vi "Get Monitor Configuration.vi"(8 "error in (no error)":errorcluster) -> (0 "error out":errorcluster, 1 "Primary Display Index":i32, 2 "Display Preview":picture, 3 "Display Areas":T1(array[cluster]))   [LabVIEW 2023]
doc: "This will return an array of clusters with the Horizontal and verticle dimensions in pixels for each display."
uses:
  <vilib>/Analysis/baseanly.llb/Mean (DBL).vi
  System.Windows.Forms
  System.Drawing
  <vilib>/Analysis/NI_AALBase.lvlib
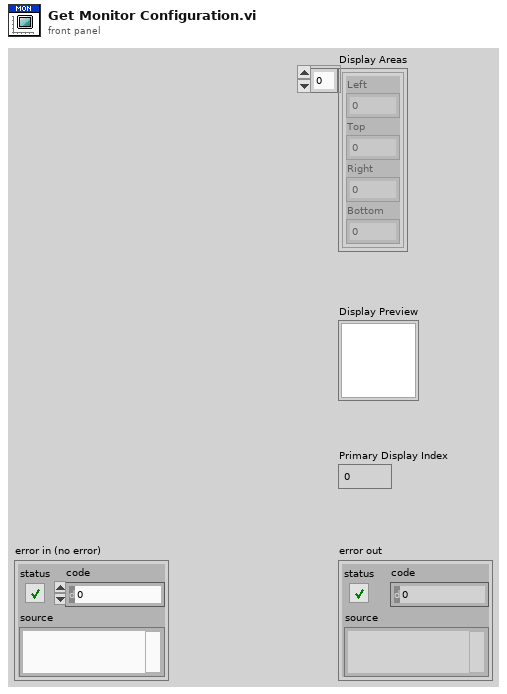
[diagram p1: front panel]
types:
  T1 = cluster{"Left":i32, "Top":i32, "Right":i32, "Bottom":i32}[]
  T2 = cluster{"horizontal":enum16{"left", "center", "right"}, "vertical":enum16{"top", "center", "bottom"}}
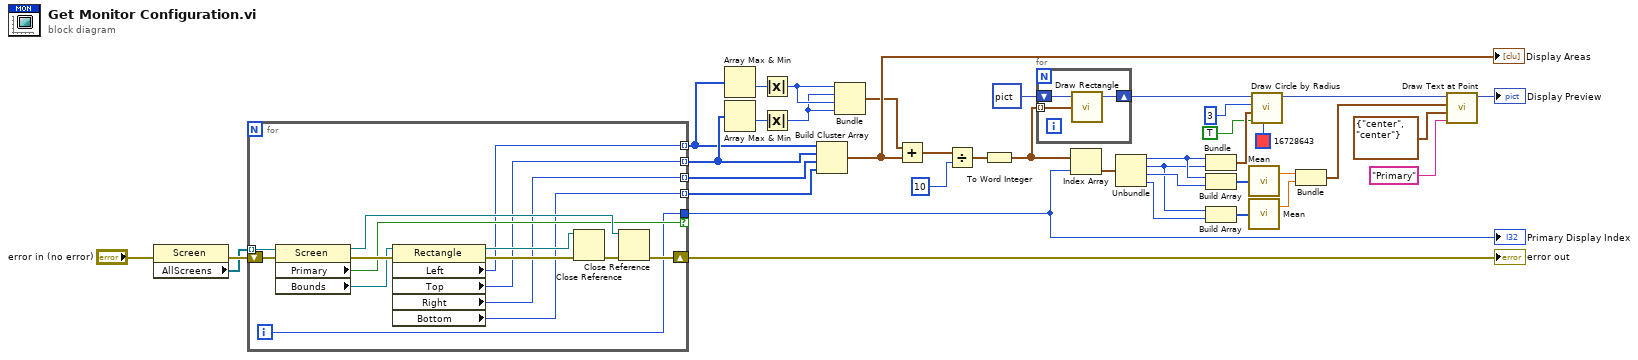
[diagram p0: block diagram]
diagram:
  n1 = property class="Screen"(error in="error in (no error)") -> (error out=w36:errorcluster, "AllScreens"=w34:refnum<k24>[])  [unwired: 1 in, 1 out]
  n2 = for {
    tunnel: w34 -> [w48] mode=indexing
    shift-right: [w46] -> w33
    shift-left: w36 -> [w49]
    tunnel: [w45] -> w6 mode=indexing
    tunnel: [w44] -> w30 mode=indexing
    tunnel: [w43] -> w32 mode=indexing
    tunnel: [w42] -> w31 mode=indexing
    tunnel: [w41] -> w20 if=w52
    i -> [w41]
    n3 = property class="Screen"(reference=w48, error in=w49) -> (reference out=w53:refnum<k24>, error out=w54:errorcluster, "Primary"=w52:bool, "Bounds"=w40:refnum<k24>)
    n4 = property class="Rectangle"(reference=w40, error in=w54) -> (reference out=w51:refnum<k24>, error out=w50:errorcluster, "Left"=w45:i32, "Top"=w44:i32, "Right"=w43:i32, "Bottom"=w42:i32)
    n5 = Close Reference(reference=w51, error in (no error)=w50) -> (error out=w47:errorcluster)
    n6 = Close Reference(reference=w53, error in (no error)=w47) -> (error out=w46:errorcluster)
  }
  "error out" <- w33
  "Primary Display Index" <- w20
  n7 = Array Max & Min(array=w6) -> (min value=w29:i32)  [unwired: 3 out]
  n8 = Array Max & Min(array=w30) -> (min value=w28:i32)  [unwired: 3 out]
  n9 = Absolute Value(x=w29) -> (abs(x)=w5:i32)
  n10 = Absolute Value(x=w28) -> (abs(x)=w4:i32)
  n11 = Build Cluster Array(w6, w30, w32, w31) -> (w3:T1)
  "Display Areas" <- w3
  n12 = Bundle(w5, w4, w5, w4) -> (w2:cluster{i32, i32, i32, i32})  [unwired: 1 in]
  n13 = Add(x=w2, y=w3) -> (x+y=w1:cluster{i32, i32, i32, i32}[])
  n14 = Divide(x=w1, y=10) -> (x/y=w21:cluster{dbl, dbl, dbl, dbl}[])
  n15 = To Word Integer(number=w21) -> (16bit integer=w19:cluster{i16, i16, i16, i16}[])
  n16 = for {
    shift-right: [w56] -> w24
    shift-left: picture data[5B] ("picture") -> [w57]
    tunnel: w19 -> [w55] mode=indexing
    n17 = call <vilib>:"Draw Rectangle.vi"("picture"=w57, "rect"=w55) -> ("new picture"=w56:picture)  [unwired: 7 in]
  }
  n18 = Index Array(array=w19, index=w20) -> (element=w18:cluster{i16, i16, i16, i16})
  n19 = Unbundle(w18) -> (w16:i16, w14:i16, w15:i16, w13:i16)
  n20 = Bundle(w16, w14) -> (w37:cluster{i16, i16})  [unwired: 1 in]
  n21 = Build Array(w16, w15) -> (w12:i16[])
  n22 = Build Array(w14, w13) -> (w11:i16[])
  n23 = call-poly <vilib>:"Mean.vi"("X"=w12) -> ("mean"=w10:dbl)  [unwired: 1 out]
  n24 = call-poly <vilib>:"Mean.vi"("X"=w11) -> ("mean"=w9:dbl)  [unwired: 1 out]
  n25 = call <vilib>:"Draw Circle by Radius.vi"("color(black)"=u32 16728643, "fill?(F)"=TRUE, "pixel center"=w37, "radius"=i16 3, "picture"=w24) -> ("new picture"=w17:picture)  [unwired: 6 in]
  n26 = Bundle("mean"=w10, "mean"=w9) -> (w8:cluster{"mean":dbl, "mean":dbl})  [unwired: 1 in]
  n27 = call <vilib>:"Draw Text at Point.vi"("text"="Primary", "alignment(left, top)"=T2 {"horizontal"=enum."center", "vertical"=enum."center"}, "origin"=w8, "picture"=w17) -> ("new picture"=→"Display Preview":picture)  [unwired: 6 in, 1 out]
